vi "RunAutoFile.vi"(8 "error in (no error)":errorcluster, 10 "AutoFile":string) -> (0 "error out":errorcluster)   [LabVIEW 2017]
uses:
  Shared/PathFileData.ctl
  Shared/RobotNeededPathData.ctl
  d3721f1b-958b-4040-9e37-572c9a7237de.vi
  e484f707-ba5e-4066-990d-529f066dd433.vi
  fc2c1253-312f-4133-ab24-205336c59347.vi
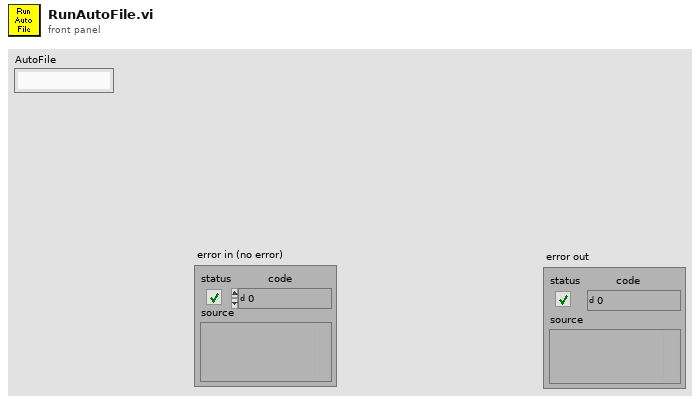
[diagram p1: front panel]
types:
  T1 = typedef "AutoFileDataType.ctl" = dbl[][]
  T2 = typedef "Command Status Info.ctl" = cluster{"Name":string, "Status":T3, "notifier out":T4}
  T3 = typedef "Completion Status.ctl" = enum16{"Successful", "Aborted", "Incomplete"}
  T4 = typedef "Completion Notifier.ctl" = refnum<notifier>
  T5 = typedef "PathFileData.ctl" = cluster{"RobotNeeded":T6, "Meta":cluster{"Path (px)":cluster{i32, i32}[], "RobotWidth":dbl, "RobotLength":dbl, "CenterOfRotYOffset":dbl, "Roundedness":dbl, "StartingPositionPreset":u32, "PathName":string}}
  T6 = typedef "RobotNeededPathData.ctl" = cluster{"Path":cluster{dbl, dbl}[], "MaxVel":dbl, "MaxAccel":dbl, "Backwards?":bool, "PointSpacing":dbl, "LookaheadDist":dbl, "Speed/Curve":dbl, "SlowDistanceAtEnd":dbl, "SlowSpeed":dbl}
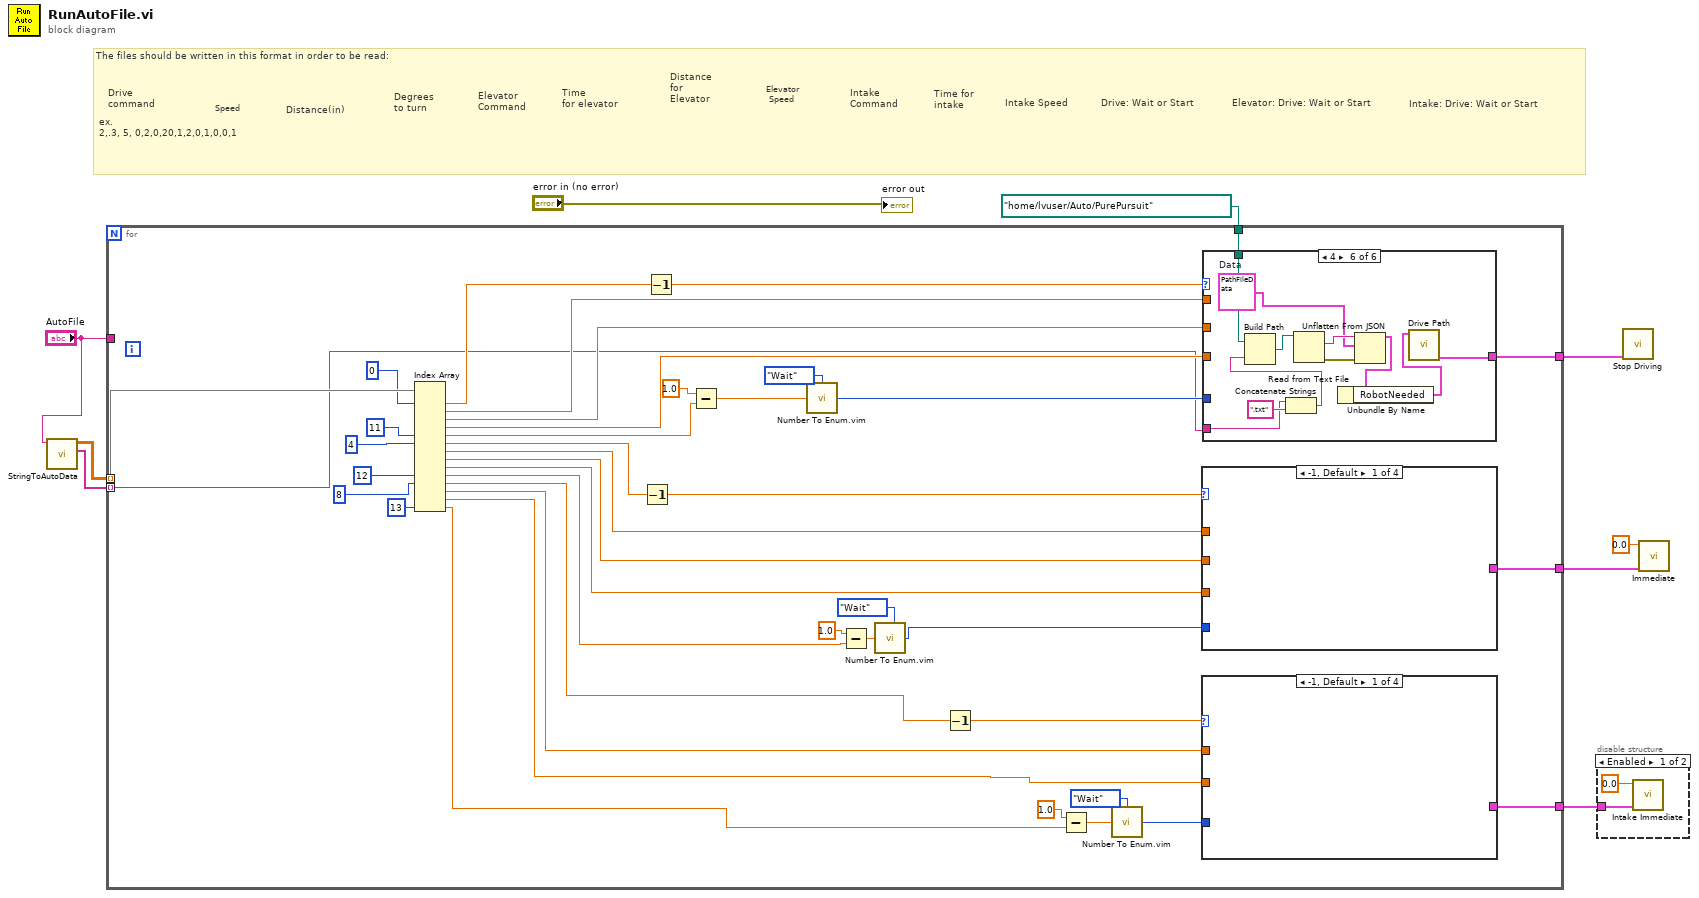
[diagram p0: block diagram]
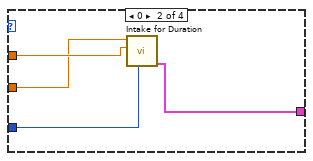
[diagram p2: hidden frame]
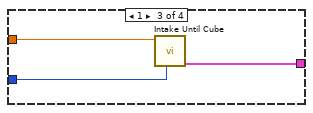
[diagram p3: hidden frame]
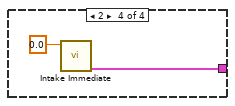
[diagram p4: hidden frame]
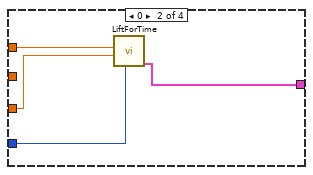
[diagram p5: hidden frame]
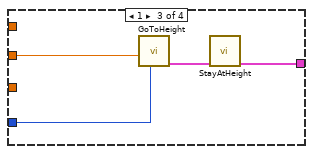
[diagram p6: hidden frame]
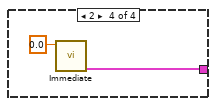
[diagram p7: hidden frame]
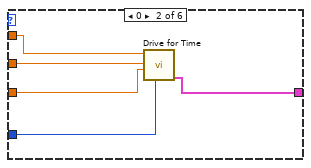
[diagram p9: hidden frame]
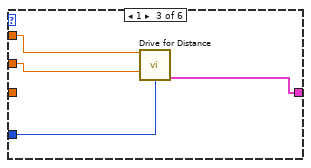
[diagram p10: hidden frame]
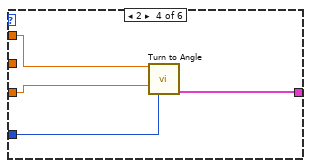
[diagram p11: hidden frame]
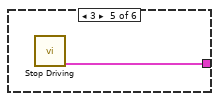
[diagram p12: hidden frame]
diagram:
  # "Intake: Drive: Wait or Start"
  # "Elevator: Drive: Wait or Start"
  # "Drive: Wait or Start"
  # "Time\nfor elevator"
  # "Intake Speed"
  # "Time for \nintake"
  # "Intake \nCommand"
  # "Elevator\n Speed"
  # "Elevator\nCommand"
  # "Distance \nfor\nElevator"
  # "Drive\ncommand"
  # "Degrees \nto turn"
  # "Distance(in)"
  # "Speed"
  # "The files should be written in this format in order to be read:\n                                                                                                                                                                                                                                                                            \n\n\n\n\n ex. \n 2,.3, 5, 0,2,0,20,1,2,0,1,0,0,1"
  n1 = call "StringToAutoData.vi"("String"="AutoFile") -> ("Path File Names"=w3:string[], "Auto"=w2:T1)  [unwired: 9 in]
  n2 = for {
    tunnel: "AutoFile" -> [_]
    tunnel: [w47] -> w7
    tunnel: [w46] -> w8
    tunnel: w2 -> [w33] mode=indexing
    tunnel: [w18] -> w5
    tunnel: w3 -> [w11] mode=indexing
    tunnel: path "/home/lvuser/Auto/PurePursuit" ("base path") -> [w10]
    n3 = Index Array(array=w33, index #1=0 ("index"), index #5=11 ("index"), index #6=4 ("index"), index #10=12 ("index"), index #11=8 ("index"), index #14=13 ("index")) -> (element #1=w32:dbl, element #2=w31:dbl, element #3=w30:dbl, element #4=w29:dbl, element #5=w28:dbl, element #6=w27:dbl, element #7=w26:dbl, element #8=w25:dbl, element #9=w24:dbl, element #10=w23:dbl, element #11=w22:dbl, element #12=w21:dbl, element #13=w20:dbl, element #14=w19:dbl)  [unwired: 8 in]
    n4 = Decrement(x=w27) -> (x-1=w49:dbl)
    n5 = Decrement(x=w32) -> (x-1=w50:dbl)
    n6 = Subtract(x=1.0, y=w28) -> (x-y=w43:dbl)
    n7 = call "Number To Enum.vim"("number"=w43, "enum type"=enum16{"Start", "Wait"}."Wait" ("Synchronization")) -> ("number as enum"=w42:enum16{"Start", "Wait"})
    n8 = Subtract(x=1.0, y=w23) -> (x-y=w41:dbl)
    n9 = call "Number To Enum.vim"("number"=w41, "enum type"=enum16{"Start", "Wait"}."Wait" ("Synchronization")) -> ("number as enum"=w38:enum16{"Start", "Wait"})
    n10 = Decrement(x=w22) -> (x-1=w48:dbl)
    n11 = Subtract(x=1.0, y=w19) -> (x-y=w36:dbl)
    n12 = call "Number To Enum.vim"("number"=w36, "enum type"=enum16{"Start", "Wait"}."Wait" ("Synchronization")) -> ("number as enum"=w34:enum16{"Start", "Wait"})
    n13 = case shown="-1, Default" w49 {
      tunnel: w26 -> [_ w63 _ _]
      tunnel: w25 -> [_ _ w66 _]
      tunnel: w24 -> [_ w62 _ _]
      tunnel: [_ w61 w65 w68] -> w46
      tunnel: w38 -> [_ w60 w64 _]
      frame -1, Default {
      }
      frame 0 {
        n14 = call "LiftForTime.vi"("Synchronization"=w60, "Setpoint"=w62, "Duration (s)"=w63) -> ("Command Info Out"=w61:T2)  [unwired: 8 in]
      }
      frame 1 {
        n15 = call "GoToHeight.vi"("Synchronization"=w64, "Setpoint"=w66) -> ("Command Info Out"=w67:T2)  [unwired: 9 in]
        n16 = call "StayAtHeight.vi"("Command Info In"=w67) -> ("Command Info Out"=w65:T2)  [unwired: 10 in]
      }
      frame 2 {
        n17 = call "Immediate.vi"("Setpoint"=0.0) -> ("Command Info Out"=w68:T2)  [unwired: 10 in]
      }
    }
    n18 = case shown="-1, Default" w48 {
      tunnel: w21 -> [_ w54 _ _]
      tunnel: w20 -> [_ w53 w57 _]
      tunnel: [_ w52 w56 w58] -> w18
      tunnel: w34 -> [_ w51 w55 _]
      frame -1, Default {
      }
      frame 0 {
        n19 = call "Intake for Duration.vi"("Synchronization"=w51, "Duration (s)"=w54, "Speed"=w53) -> ("Command Info Out"=w52:T2)  [unwired: 8 in]
      }
      frame 1 {
        n20 = call "Intake Until Cube.vi"("Synchronization"=w55, "Speed"=w57) -> ("Command Info Out"=w56:T2)  [unwired: 9 in]
      }
      frame 2 {
        n21 = call "Intake Immediate.vi"("Speed"=0.0 ("Setpoint")) -> ("Command Info Out"=w58:T2)  [unwired: 10 in]
      }
    }
    n22 = case shown="4" w50 {
      tunnel: w31 -> [_ w74 w78 w82 _ _]
      tunnel: w30 -> [_ w73 w77 _ _ _]
      tunnel: w29 -> [_ w72 _ w81 _ _]
      tunnel: [_ w71 w76 w80 w83 w87] -> w47
      tunnel: w42 -> [_ w70 w75 w79 _ _]
      tunnel: w11 -> [_ _ _ _ _ w88]
      tunnel: w10 -> [_ _ _ _ _ w89]
      frame -1, Default {
      }
      frame 0 {
        n23 = call "Drive for Time.vi"("Synchronization"=w70, "Seconds"=w72, "Right Speed"=w73, "Left Speed"=w74) -> ("Command Info Out"=w71:T2)  [unwired: 6 in, 1 out]
      }
      frame 1 {
        n24 = call "Drive for Distance.vi"("Speed"=w78, "Distance (inch)"=w77, "Synchronication"=w75) -> ("Command Info Out"=w76:T2)  [unwired: 12 in]
      }
      frame 2 {
        n25 = call "Turn to Angle.vi"("Speed"=w82, "Target Angle"=w81, "Synchronication"=w79) -> ("Command Info Out"=w80:T2)  [unwired: 12 in]
      }
      frame 3 {
        n26 = call "Stop Driving.vi"() -> ("Command Info Out"=w83:T2)  [unwired: 11 in]
      }
      frame 4 {
        w85 = T5 {"RobotNeeded"={"Path"=[], "MaxVel"=0.0, "MaxAccel"=0.0, "Backwards?"=FALSE, "PointSpacing"=0.0, "LookaheadDist"=0.0, "Speed/Curve"=1.8, "SlowDistanceAtEnd"=12.0, "SlowSpeed"=15.0}, "Meta"={"Path (px)"=[], "RobotWidth"=0.0, "RobotLength"=0.0, "CenterOfRotYOffset"=0.0, "Roundedness"=0.0, "StartingPositionPreset"=0, "PathName"=""}}  # Data
        n27 = Concatenate Strings(w88, ".txt" ("string")) -> (w94:string)
        n28 = Build Path(base path=w89, name or relative path=w94) -> (appended path=w93:path)
        n29 = Read from Text File(file (use dialog)=w93) -> (text=w91:string, error out=w92:errorcluster)  [unwired: 3 in, 2 out]
        n30 = Unflatten From JSON(JSON string=w91, type and defaults=w85, error in (no error)=w92) -> (value=w86:T5)  [unwired: 4 in, 1 out]
        n31 = Unbundle By Name(w86) -> ("RobotNeeded"=w84:T6)
        n32 = call "Drive Path.vi"("Path"=w84) -> ("Command Info Out"=w87:T2)  [unwired: 10 in]
      }
    }
  }
  n33 = disable-structure shown="Enabled" {
    disable-tunnel: w5 -> [w95 _]
    frame Enabled {
      n34 = call "Intake Immediate.vi"("Command Info In"=w95, "Speed"=0.0 ("Setpoint")) -> ()  [unwired: 9 in, 1 out]
    }
    frame Disabled {
    }
  }
  n35 = call "Stop Driving.vi"("Command Info In"=w7) -> ()  [unwired: 10 in, 1 out]
  n36 = call "Immediate.vi"("Command Info In"=w8, "Setpoint"=0.0) -> ()  [unwired: 9 in, 1 out]
  "error out" <- "error in (no error)"
